vi "读取数据库.vi"(5 "精度(6)":i16=2, 7 "condition":string, 8 "error in (no error)":errorcluster caption="错误输入（无错误）", 9 "database":string="database1.mdb", 10 "显示项":string[](array[string]), 11 "组合框":string(combo)) -> (0 "error out":errorcluster caption="错误输出", 1 "columns":string[](array[string]), 2 "data":variant[][](array[variant]), 3 "表格":string[][](table))   [LabVIEW 2016]
uses:
  <vilib>/Utility/sysdir.llb/System Directory Type.ctl
  <vilib>/addons/database/Connection.llb/DB Tools Open Connec (String).vi
  <vilib>/addons/database/_DB Variant To Data/Database Variant To Data.xnode
  <vilib>/addons/database/NI_Database_API.lvlib
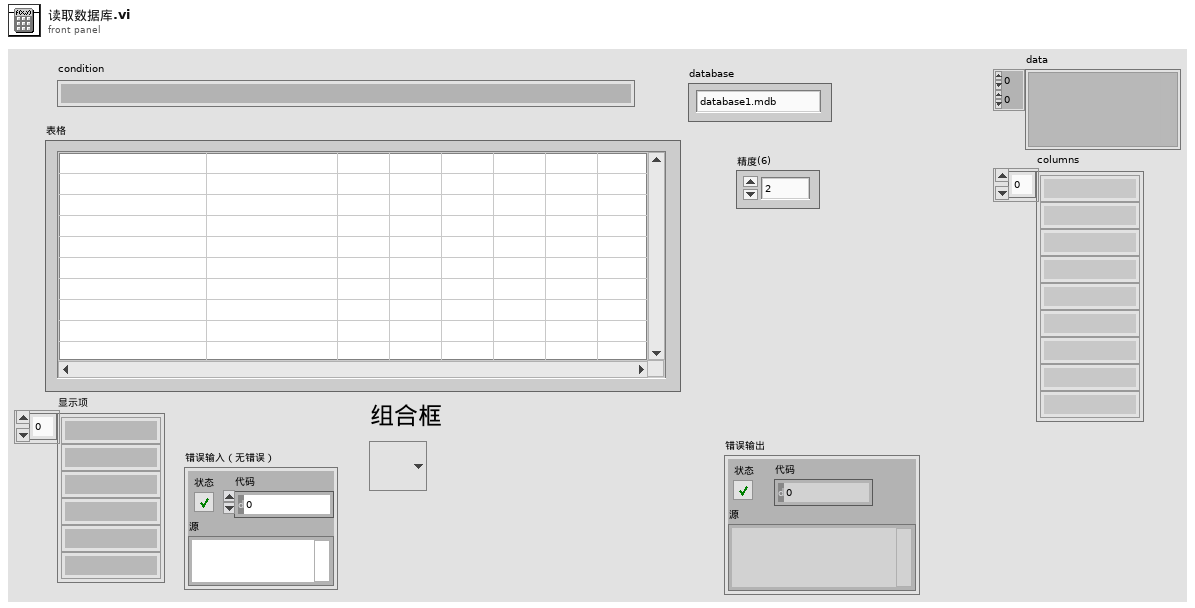
[diagram p1: front panel]
types:
  T1 = typedef "System Directory Type.ctl" = i32
  T2 = typedef "NI_Database_API.lvlib/Conn ObjectReference.ctl" = refnum<k1>
  T3 = typedef "NI_Database_API.lvlib/DB Tools DataTypes.ctl" = enum16{"String", "Long (I32)", "Single (SGL)", "Double (DBL)", "Date/Time", "Binary"}
  T4 = cluster{"name":string, "database data type":T3, "defined size":i32}[]
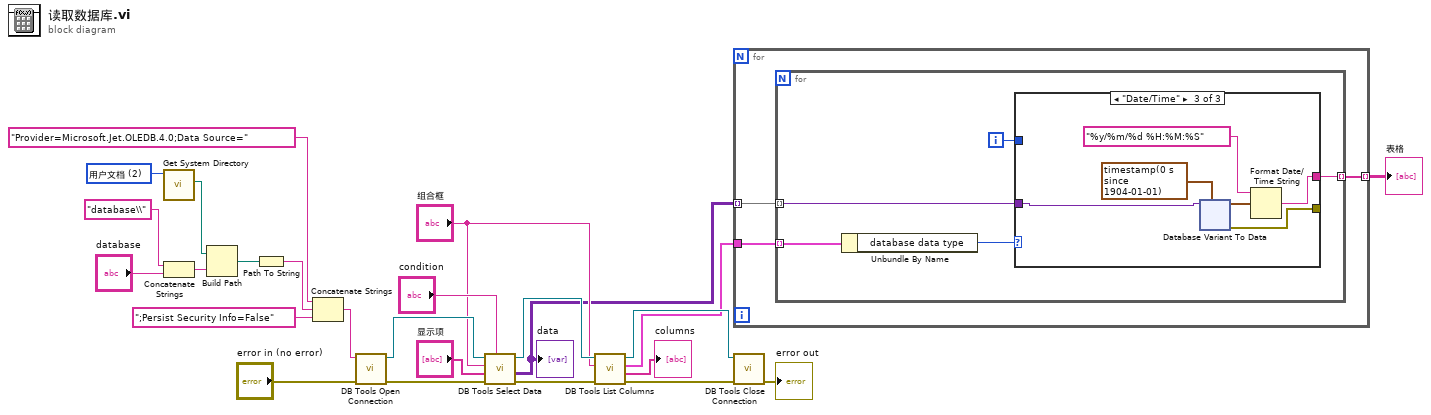
[diagram p0: block diagram]
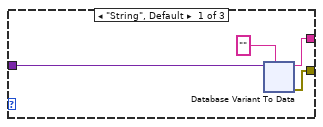
[diagram p2: hidden frame]
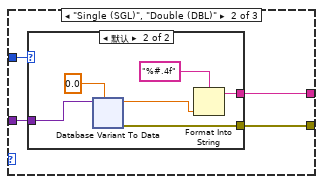
[diagram p3: hidden frame]
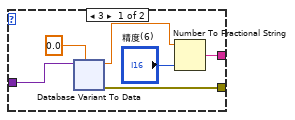
[diagram p4: hidden frame]
diagram:
  w10 = T1 2 items=["用户目录"=0, "用户桌面"=1, "用户文档"=2, "用户应用程序数据"=3, "用户设置"=4, "用户临时目录"=5, "公共文档"=6, "公共应用程序数据"=7, "公共设置"=8, "公共缓存"=13, "系统核心库"=9, "系统安装库"=10, "应用程序文件"=11, "启动盘根目录"=12] ("system directory type")
  n1 = call <vilib>:"Get System Directory.vi"("system directory type"=w10) -> ("system directory"=w9:path)  [unwired: 10 in]
  n2 = Concatenate Strings("database\\" ("名称或相对路径"), "database") -> (w6:string)
  n3 = Build Path(base path=w9, name or relative path=w6) -> (appended path=w11:path)
  n4 = Path To String(path=w11) -> (string=w12:string)
  n5 = Concatenate Strings("Provider=Microsoft.Jet.OLEDB.4.0;Data Source=", w12, ";Persist Security Info=False") -> (w8:string)
  n6 = call-poly <vilib>:"DB Tools Open Connection.vi"("error in (no error)"="error in (no error)", "connection information"=w8) -> ("error out"=w24:errorcluster, "connection reference"=w25:T2)  [unwired: 6 in]
  n7 = call <vilib>:"DB Tools Select Data.vi"("condition"="condition", "error in (no error)"=w24, "columns"="显示项", "table"="组合框", "connection reference"=w25) -> ("error out"=w23:errorcluster, "data"=w3:variant[][], "connection reference out"=w20:T2)  [unwired: 1 in]
  "data" <- w3
  n8 = call <vilib>:"DB Tools List Columns.vi"("error in (no error)"=w23, "table"="组合框", "connection reference"=w20) -> ("error out"=w15:errorcluster, "columns"=→"columns":string[], "column information"=w2:T4, "connection reference out"=w16:T2)  [unwired: 1 in]
  n9 = for {
    tunnel: w3 -> [w28] mode=indexing
    tunnel: w2 -> [w27]
    tunnel: [w26] -> w1 mode=indexing
    n10 = for {
      tunnel: w28 -> [w32] mode=indexing
      tunnel: w27 -> [w31] mode=indexing
      tunnel: [w29] -> w26 mode=indexing
      i -> [w30]
      n11 = Unbundle By Name(w31) -> ("database data type"=w33:T3)
      n12 = case shown="\"Date/Time\"" w33 {
        tunnel: w32 -> [w37 w73 w155]
        tunnel: [w36 w72 w151] -> w29
        tunnel: w30 -> [_ w71 _]
        tunnel: [w34 w70 w150] -> _
        frame "String", Default {
          n13 = xnode "Database Variant To Data"("database variant"=w37, "type"="") -> ("data"=w36:string, "error out"=w34:errorcluster)  [unwired: 1 in]
        }
        frame "Single (SGL)", "Double (DBL)" {
          n14 = case shown="默认" w71 {
            tunnel: w73 -> [w79 w117]
            tunnel: [w77 w115] -> w72
            tunnel: [w74 w112] -> w70
            frame 3 {
              n15 = xnode "Database Variant To Data"("database variant"=w79, "type"=0.0) -> ("data"=w78:dbl, "error out"=w74:errorcluster)  [unwired: 1 in]
              n16 = Number To Fractional String(number=w78, precision (6)="精度(6)") -> (F-format string=w77:string)  [unwired: 2 in]
            }
            frame Default {
              n17 = xnode "Database Variant To Data"("database variant"=w117, "type"=0.0) -> ("data"=w116:dbl, "error out"=w112:errorcluster)  [unwired: 1 in]
              n18 = Format Into String(format string="%#.4f" ("格式字符串"), w116) -> (resulting string=w115:string)  [unwired: 2 in, 1 out]
            }
          }
        }
        frame "Date/Time" {
          n19 = xnode "Database Variant To Data"("database variant"=w155, "type"=timestamp(0 s since 1904-01-01) ("当前时间")) -> ("data"=w154:timestamp, "error out"=w150:errorcluster)  [unwired: 1 in]
          n20 = Format Date/Time String(time format string (%c)="%y/%m/%d %H:%M:%S" ("时间格式字符串(%c)"), seconds (now)=w154) -> (date/time string=w151:string)  [unwired: 1 in]
        }
      }
    }
  }
  "表格" <- w1
  n21 = call <vilib>:"DB Tools Close Connection.vi"("error in (no error)"=w15, "connection reference"=w16) -> ("error out"=→"error out":errorcluster)  [unwired: 5 in]
